vi "High Resolution Timing.vi"(2 "relative seconds (NaN)":dbl=nan, 3 "Error In":errorcluster) -> (10 "relative seconds":dbl, 16 "elapsed (relative) seconds":dbl, 17 "Error Out":errorcluster)   [LabVIEW 2019]
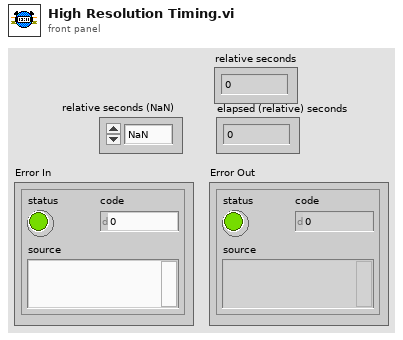
[diagram p1: front panel]
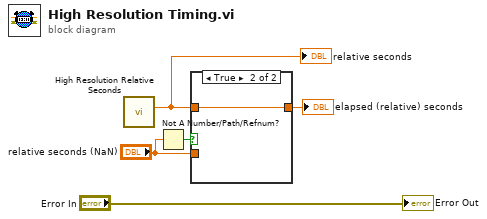
[diagram p0: block diagram]
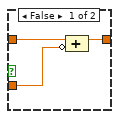
[diagram p2: hidden frame]
diagram:
  n1 = call <vilib>:"High Resolution Relative Seconds.vi"() -> ("relative seconds"=w1:dbl)
  "relative seconds" <- w1
  n2 = Not A Number/Path/Refnum?(number/path/refnum="relative seconds (NaN)") -> (NaN/Path/Refnum?=w3:bool)
  n3 = case shown="True" w3 {
    tunnel: "relative seconds (NaN)" -> [w8 _]
    tunnel: [w7 w9] -> w5
    tunnel: w1 -> [w6 w9]
    frame False {
      n4 = Compound Arithmetic op=ADD(w6, invert w8) -> (w7:dbl)
    }
    frame True {
    }
  }
  "elapsed (relative) seconds" <- w5
  "Error Out" <- "Error In"
